vi "LVClass_DataServer ctor.vi"(0 "DataServer":refnum<class "DataServer.lvclass">, 5 "config_file_path":path, 7 "port":u16, 11 "error in (no error)":errorcluster) -> (4 "DataServer out":refnum<class "DataServer.lvclass">, 15 "error out":errorcluster)   [LabVIEW 2020, in "DataServer.lvclass"]
doc: "Server constructor from configuration file and port.\n\n--------------------------------------------------------------------------------\n\n<B>serverIn </B> : Constant Pointer to server object.\n<B>serverOut </B> : Constant Pointer to server object.\n<B>config_file_path </B> : Absolute path to haso configuration file.\n<B>port </B> : Port value.\n<B>ErrorIn </B> : Error\n<B>ErrorOut </B> : Error\n\n--------------------------------------------------------------------------------"
uses:
  DataServer.lvclass
  Handle creation.ctl
  DataServer.lvclass/DataServer.ctl
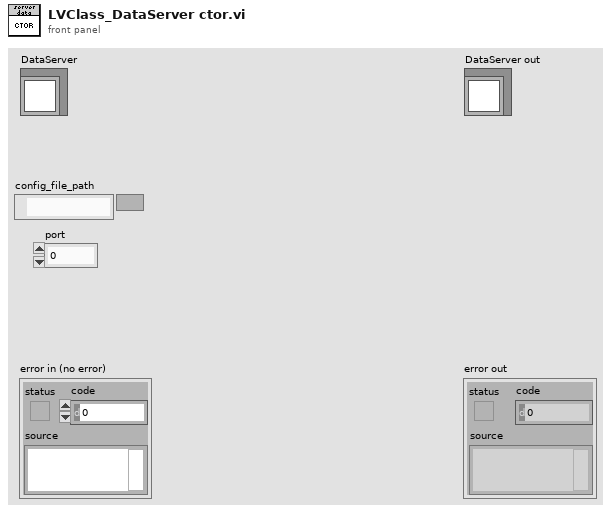
[diagram p1: front panel]
types:
  T1 = typedef "Handle creation.ctl" = enum16{"By ctor", "By write function"}
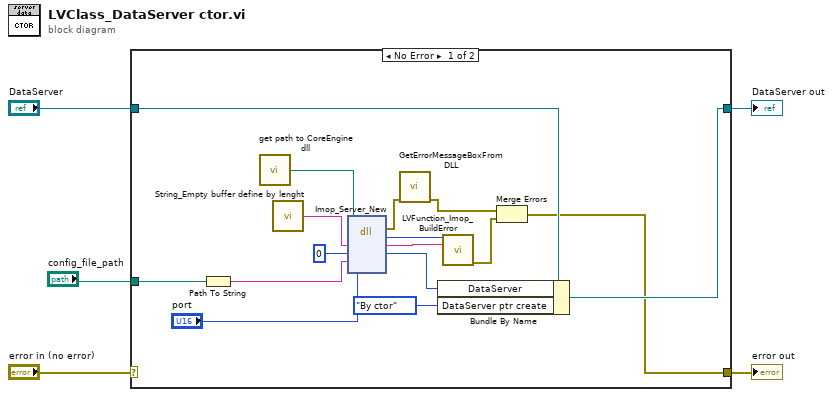
[diagram p0: block diagram]
diagram:
  n1 = case shown="No Error" "error in (no error)" {
    selector: "error in (no error)" -> [_ w23]
    tunnel: [w6 w23] -> w4
    tunnel: [w10 w22] -> w2
    tunnel: "DataServer" -> [w11 w22]
    tunnel: "config_file_path" -> [w8 _]
    frame No Error {
      n2 = Path To String(path=w8) -> (string=w9:string)
      n3 = call "get path to CoreEngine dll.vi"() -> ("path to c_interface_vc100.dll"=w16:path)  [unwired: 12 in, 3 out]
      n4 = call "String_Empty buffer define by lenght.vi"() -> ("Empty buffer"=w19:string)  [unwired: 1 in]
      n5 = dll-call lib="D:/soft/HASO_v3/SVN_trunk/ImOpCoreEngine4_LV2011/DLLs/c_interface_vc100.dll" fn="Imop_Server_New"(path in=w16, "message"=w19, "Slopes Server"=0 ("Image compat"), "path"=w9, "port"="port") -> (error out=w15:errorcluster, "return type"=w20:i32, "message"=w21:string, "Slopes Server"=w18:i32)  [unwired: 4 in, 1 out]
      n6 = call "GetErrorMessageBoxFromDLL.vi"("error IN"=w15) -> ("error OUT"=w13:errorcluster)  [unwired: 10 in]
      n7 = Bundle By Name(cluster=w11, "DataServer"=w18, "DataServer ptr create"=Handle_creation."By ctor" ("Image Compat ptr create")) -> (w10:refnum<class "DataServer.lvclass">)
      n8 = call "LVFunction_Imop_BuildError.vi"("code"=w20, "String to Prepend to source (\"\")"=w21) -> ("error out"=w12:errorcluster)  [unwired: 13 in]
      n9 = Merge Errors(w13, w12) -> (w6:errorcluster)
    }
    frame Error {
    }
  }
  "error out" <- w4
  "DataServer out" <- w2
